vi "angleBetweenTwoLines.vi"(8 "error in (no error)":errorcluster, 9 "Angle type":string(combo)="theta", 10 "Line2":T2 {"Point 2"."Y" format="%.2f"; "Point 2"."X" format="%.2f"; "Point 1"."Y" format="%.2f"; "Point 1"."X" format="%.2f"}, 11 "Line1":T2 {"Point 2"."Y" format="%.2f"; "Point 2"."X" format="%.2f"; "Point 1"."Y" format="%.2f"; "Point 1"."X" format="%.2f"}) -> (0 "error out":errorcluster, 2 "value":dbl, 3 "Angle":T1={"Point 1"={"X"=0.0, "Y"=0.0}, "Point 2"={"X"=0.0, "Y"=0.0}, "vertex"={"X"=0.0, "Y"=0.0}, "Point 1a"={"X"=0.0, "Y"=0.0}, "Point 2a"={"X"=0.0, "Y"=0.0}, "line1Point1"={"X"=0.0, "Y"=0.0}, "line1Point2"={"X"=0.0, "Y"=0.0}, "line2Point1"={"X"=0.0, "Y"=0.0}, "line2Point2"={"X"=0.0, "Y"=0.0}, "Angle type"="theta"})   [LabVIEW 2015]
uses:
  <vilib>/vision/NI_Vision_Development_Module.lvlib
panel:
  out "Angle 2":dbl format="%.2f"
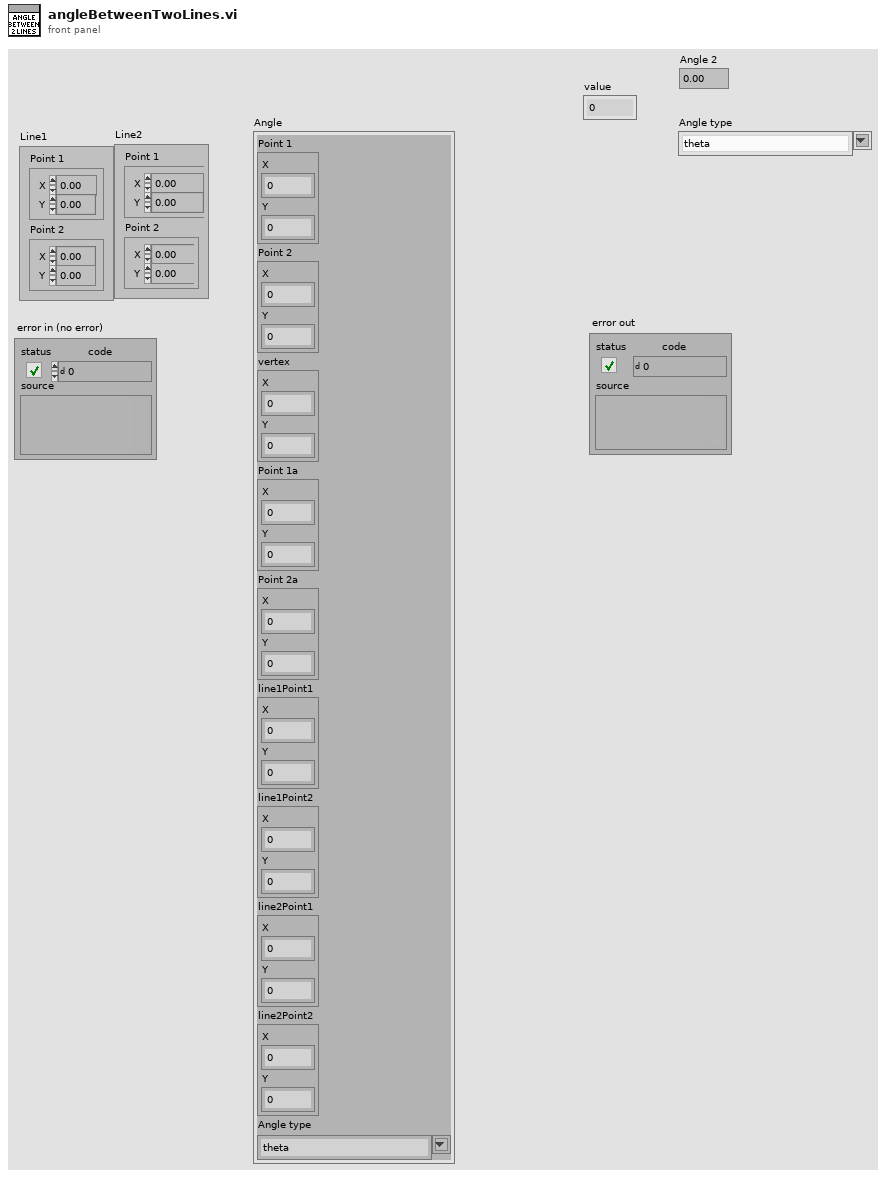
[diagram p1: front panel]
types:
  T1 = cluster{"Point 1":cluster{"X":sgl, "Y":sgl}, "Point 2":cluster{"X":sgl, "Y":sgl}, "vertex":cluster{"X":sgl, "Y":sgl}, "Point 1a":cluster{"X":sgl, "Y":sgl}, "Point 2a":cluster{"X":sgl, "Y":sgl}, "line1Point1":cluster{"X":sgl, "Y":sgl}, "line1Point2":cluster{"X":sgl, "Y":sgl}, "line2Point1":cluster{"X":sgl, "Y":sgl}, "line2Point2":cluster{"X":sgl, "Y":sgl}, "Angle type":string}
  T2 = cluster{"Point 1":cluster{"X":sgl, "Y":sgl}, "Point 2":cluster{"X":sgl, "Y":sgl}}
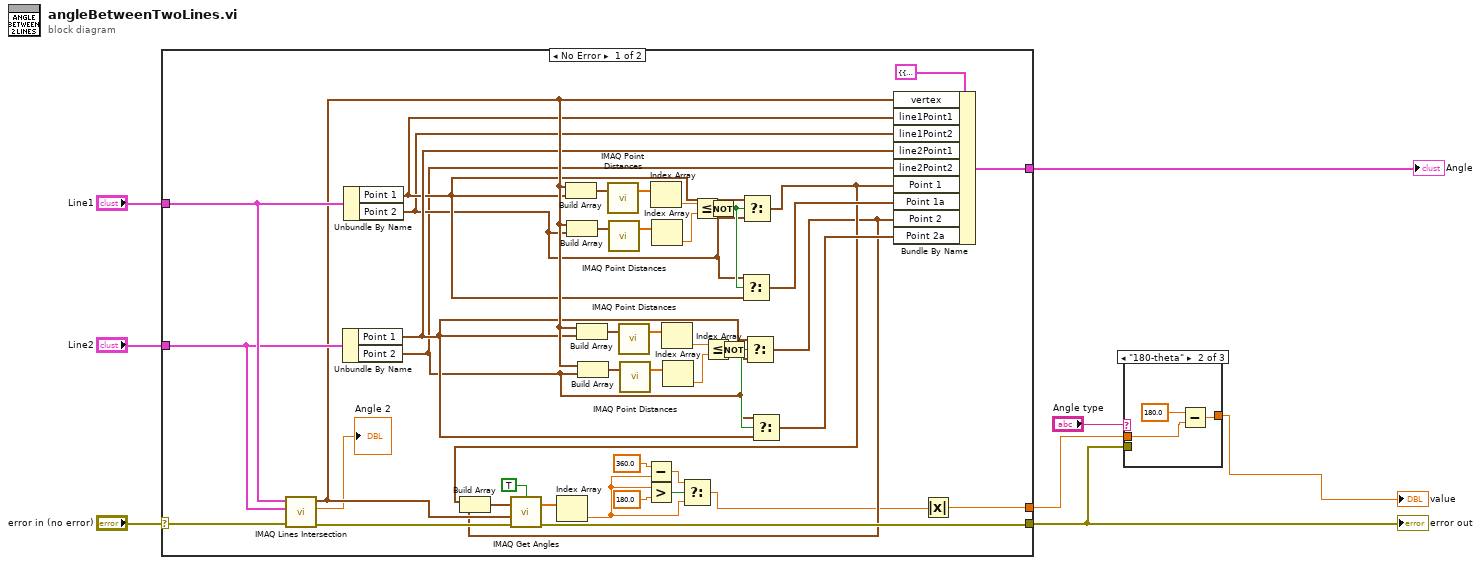
[diagram p0: block diagram]
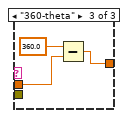
[diagram p3: hidden frame]
diagram:
  n1 = case shown="No Error" "error in (no error)" {
    selector: "error in (no error)" -> [w51 w52]
    tunnel: [w47 w52] -> w3
    tunnel: "Line1" -> [w50 _]
    tunnel: "Line2" -> [w49 _]
    tunnel: [w9 _] -> w2
    tunnel: [w18 _] -> w5
    frame No Error {
      n2 = call "IMAQ Lines Intersection"("error in (no error)"=w51, "Line 2"=w49, "Line 1"=w50) -> ("error out"=w48:errorcluster, "Angle"=→"Angle 2":dbl, "Intersection Point"=w25:cluster{"X":sgl, "Y":sgl})  [unwired: 6 in]
      n3 = Unbundle By Name(w49) -> ("Point 1"=w20:cluster{"X":sgl, "Y":sgl}, "Point 2"=w14:cluster{"X":sgl, "Y":sgl})
      n4 = Unbundle By Name(w50) -> ("Point 1"=w19:cluster{"X":sgl, "Y":sgl}, "Point 2"=w15:cluster{"X":sgl, "Y":sgl})
      n5 = Build Array(w25, w19) -> (w37:cluster{"X":sgl, "Y":sgl}[])
      n6 = Build Array(w25, w15) -> (w34:cluster{"X":sgl, "Y":sgl}[])
      n7 = Build Array(w25, w20) -> (w26:cluster{"X":sgl, "Y":sgl}[])
      n8 = Build Array(w25, w14) -> (w29:cluster{"X":sgl, "Y":sgl}[])
      n9 = call "IMAQ Point Distances"("Points"=w37) -> ("Distances"=w36:sgl[])  [unwired: 4 in, 1 out]
      n10 = call "IMAQ Point Distances"("Points"=w34) -> ("Distances"=w35:sgl[])  [unwired: 4 in, 1 out]
      n11 = call "IMAQ Point Distances"("Points"=w26) -> ("Distances"=w27:sgl[])  [unwired: 4 in, 1 out]
      n12 = call "IMAQ Point Distances"("Points"=w29) -> ("Distances"=w28:sgl[])  [unwired: 4 in, 1 out]
      n13 = Index Array(array=w36) -> (element=w33:sgl)  [unwired: 1 in]
      n14 = Index Array(array=w35) -> (element=w32:sgl)  [unwired: 1 in]
      n15 = Index Array(array=w27) -> (element=w30:sgl)  [unwired: 1 in]
      n16 = Index Array(array=w28) -> (element=w31:sgl)  [unwired: 1 in]
      n17 = Less Or Equal?(x=w33, y=w32) -> (x <= y?=w24:bool)
      n18 = Less Or Equal?(x=w30, y=w31) -> (x <= y?=w23:bool)
      n19 = Not(x=w24) -> (.not. x?=w17:bool)
      n20 = Not(x=w23) -> (.not. x?=w16:bool)
      n21 = Select(t=w15, s=w17, f=w19) -> (s? t:f=w22:cluster{"X":sgl, "Y":sgl})
      n22 = Select(t=w19, s=w17, f=w15) -> (s? t:f=w12:cluster{"X":sgl, "Y":sgl})
      n23 = Select(t=w20, s=w16, f=w14) -> (s? t:f=w11:cluster{"X":sgl, "Y":sgl})
      n24 = Build Array(w12, w11) -> (w45:cluster{"X":sgl, "Y":sgl}[])
      n25 = call "IMAQ Get Angles"("error in (no error)"=w48, "Vertex"=w25, "Points"=w45, "Use Vertex (No)"=TRUE) -> ("error out"=w47:errorcluster, "Angles (deg)"=w44:sgl[])  [unwired: 1 in, 1 out]
      n26 = Index Array(array=w44) -> (element=w39:sgl)  [unwired: 1 in]
      n27 = Subtract(x=360.0, y=w39) -> (x-y=w40:dbl)
      n28 = Greater?(x=w39, y=sgl 180.0) -> (0:w43:bool)
      n29 = Select(t=w40, s=w43, f=w39) -> (s? t:f=w10:dbl)
      n30 = Select(t=w14, s=w16, f=w20) -> (s? t:f=w21:cluster{"X":sgl, "Y":sgl})
      n31 = Bundle By Name(cluster=T1 {"Point 1"={"X"=0.0, "Y"=0.0}, "Point 2"={"X"=0.0, "Y"=0.0}, "vertex"={"X"=0.0, "Y"=0.0}, "Point 1a"={"X"=0.0, "Y"=0.0}, "Point 2a"={"X"=0.0, "Y"=0.0}, "line1Point1"={"X"=0.0, "Y"=0.0}, "line1Point2"={"X"=0.0, "Y"=0.0}, "line2Point1"={"X"=0.0, "Y"=0.0}, "line2Point2"={"X"=0.0, "Y"=0.0}, "Angle type"="theta"} ("Angle"), "vertex"=w25, "line1Point1"=w19, "line1Point2"=w15, "line2Point1"=w20, "line2Point2"=w14, "Point 1"=w12, "Point 1a"=w22, "Point 2"=w11, "Point 2a"=w21) -> (w18:T1)
      n32 = Absolute Value(x=w10) -> (abs(x)=w9:dbl)
    }
    frame Error {
    }
  }
  "error out" <- w3
  "Angle" <- w5
  n33 = case shown="\"180-theta\"" "Angle type" {
    tunnel: w3 -> [_ _ _]
    tunnel: [w53 w54 w57] -> w1
    tunnel: w2 -> [w53 w55 w58]
    frame "theta", Default {
    }
    frame "180-theta" {
      n34 = Subtract(x=180.0, y=w55) -> (x-y=w54:dbl)
    }
    frame "360-theta" {
      n35 = Subtract(x=360.0, y=w58) -> (x-y=w57:dbl)
    }
  }
  "value" <- w1
